vi "Initialization.vi"(6 "Skip Loading?":bool, 7 "Model Name":T3, 8 "Error In":errorcluster, 9 "Intialize?":bool=TRUE, 10 "Inputs":T1, 11 "Start SM":dbl=100.0 format="%#_13g") -> (0 "error out":errorcluster, 1 "Completed":bool, 4 "Status":cluster{"Status":string, "Elapsed Time":dbl}, 5 "Waveform Graph":dbl[][](graph))   [LabVIEW 2017]
doc: "Changelog:\n\n------------\nv0.1:\n- Bypass sensor 1 for all front\n\nv0.1:\n- Start Travel time taken from when the start moving command is given (previous state)\n- Total travel time is taken until the movement is stopped"
uses:
  controls/Model Name.ctl
  controls/All Inputs.ctl
  controls/SACB DI.ctl
  controls/Initialization.ctl
  controls/FGV DO.ctl
panel:
  in  "Stall Time":u32=100
  out "Graph":dbl[][](array[numeric])
  in  "Delay (for Rest)":u32=100
  in  "Timeout (ms)":u32=45000
  # "Inputs"
  # "Variables"
  # "Outputs"
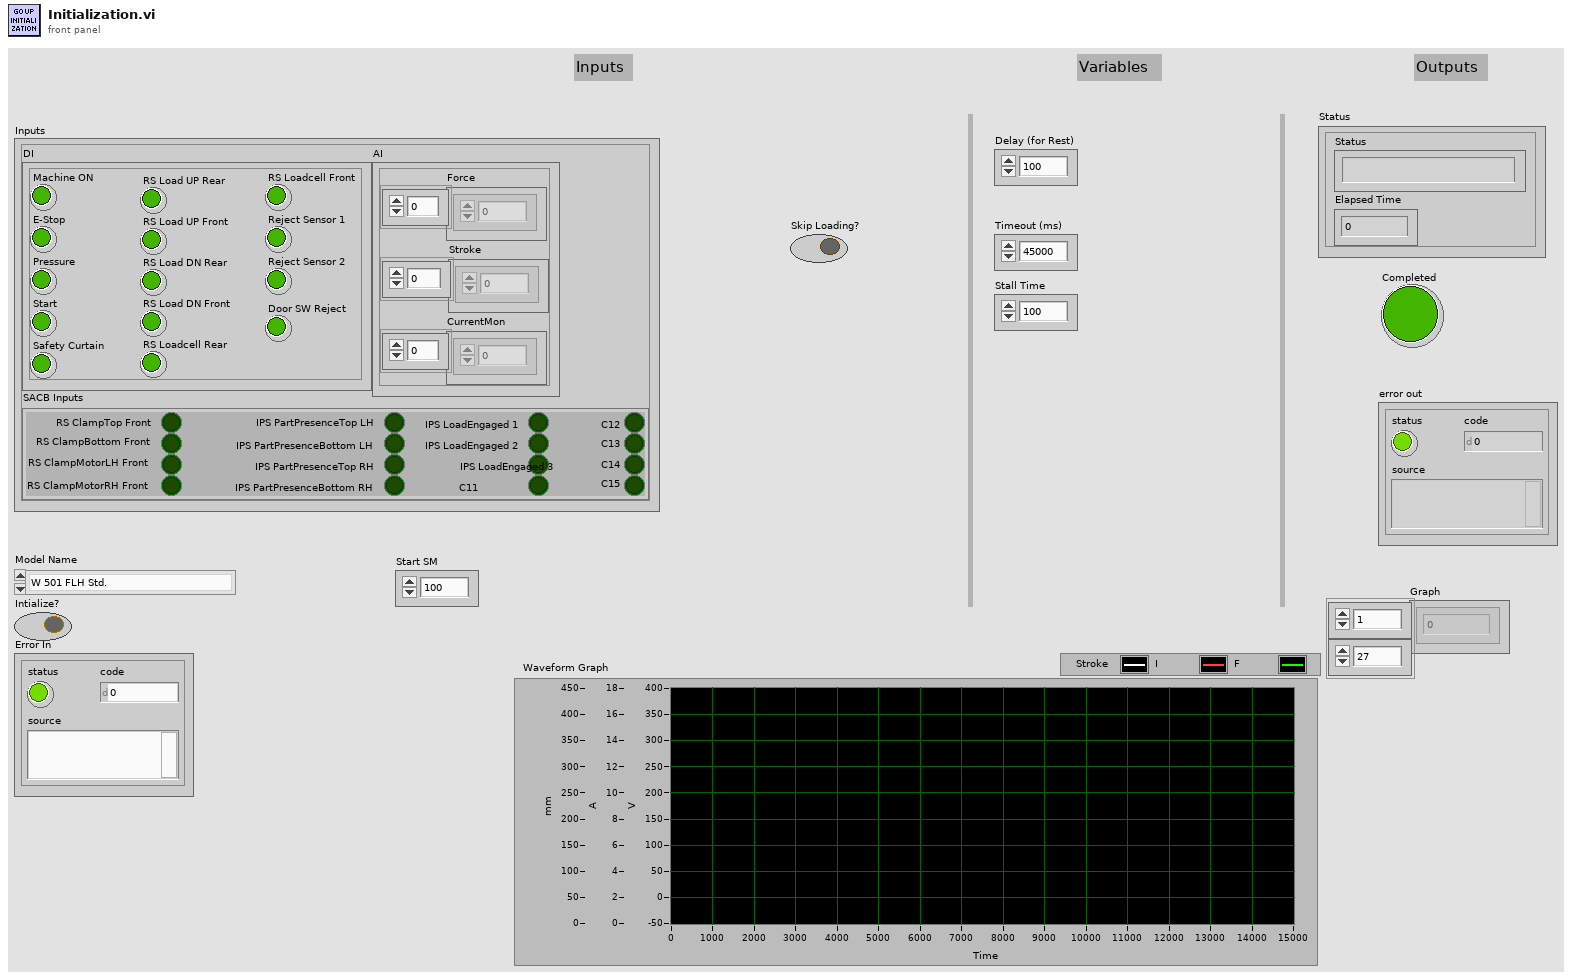
[diagram p1: front panel]
types:
  T1 = typedef "All Inputs.ctl" = cluster{"DI":cluster{"Machine ON":bool, "E-Stop":bool, "Pressure":bool, "Start":bool, "Safety Curtain":bool, "RS Load UP Rear":bool, "RS Load UP Front":bool, "RS Load DN Rear":bool, "RS Load DN Front":bool, "RS Loadcell Rear":bool, "RS Loadcell Front":bool, "Reject Sensor 1":bool, "Reject Sensor 2":bool, "Door SW Reject":bool}, "AI":cluster{"Force":dbl[], "Stroke":dbl[], "CurrentMon":dbl[]}, "SACB Inputs":T2}
  T2 = typedef "SACB DI.ctl" = cluster{"RS ClampTop Front":bool, "RS ClampBottom Front":bool, "RS ClampMotorLH Front":bool, "RS ClampMotorRH Front":bool, "IPS PartPresenceTop LH":bool, "IPS PartPresenceBottom LH":bool, "IPS PartPresenceTop RH":bool, "IPS PartPresenceBottom RH":bool, "IPS LoadEngaged 1":bool, "IPS LoadEngaged 2":bool, "IPS LoadEngaged 3":bool, "C11":bool, "C12":bool, "C13":bool, "C14":bool, "C15":bool}
  T3 = typedef "Model Name.ctl" = enum16{"W 501 FLH Std.", "W 501 FRH Std.", "W 601 FR RH Std", "W 601 FR LH Std", "W 601 RR RH Std", "W 601 RR LH Std", "W 601 FR RH AP", "W 601 FR LH AP", "W 601 RR RH AP", "W 601 RR LH AP"}
  T4 = typedef "Initialization.ctl" = enum16{"Initialize", "Check SM Position", "Check Bottom Position", "Go UP", "Check for Stall", "Turn Off Supply", "Wait for Rest", "Stall for 1s", "Turn off Supply 2", "Wait for BDC", "Done", "Error"}
  T5 = typedef "FGV DO.ctl" = enum16{"Initialize", "Start Task", "Clamping", "Load CYL", "Contactors", "Loadcell CYL", "BSL", "Read DO", "Clear Tasks", "Clear Task"}
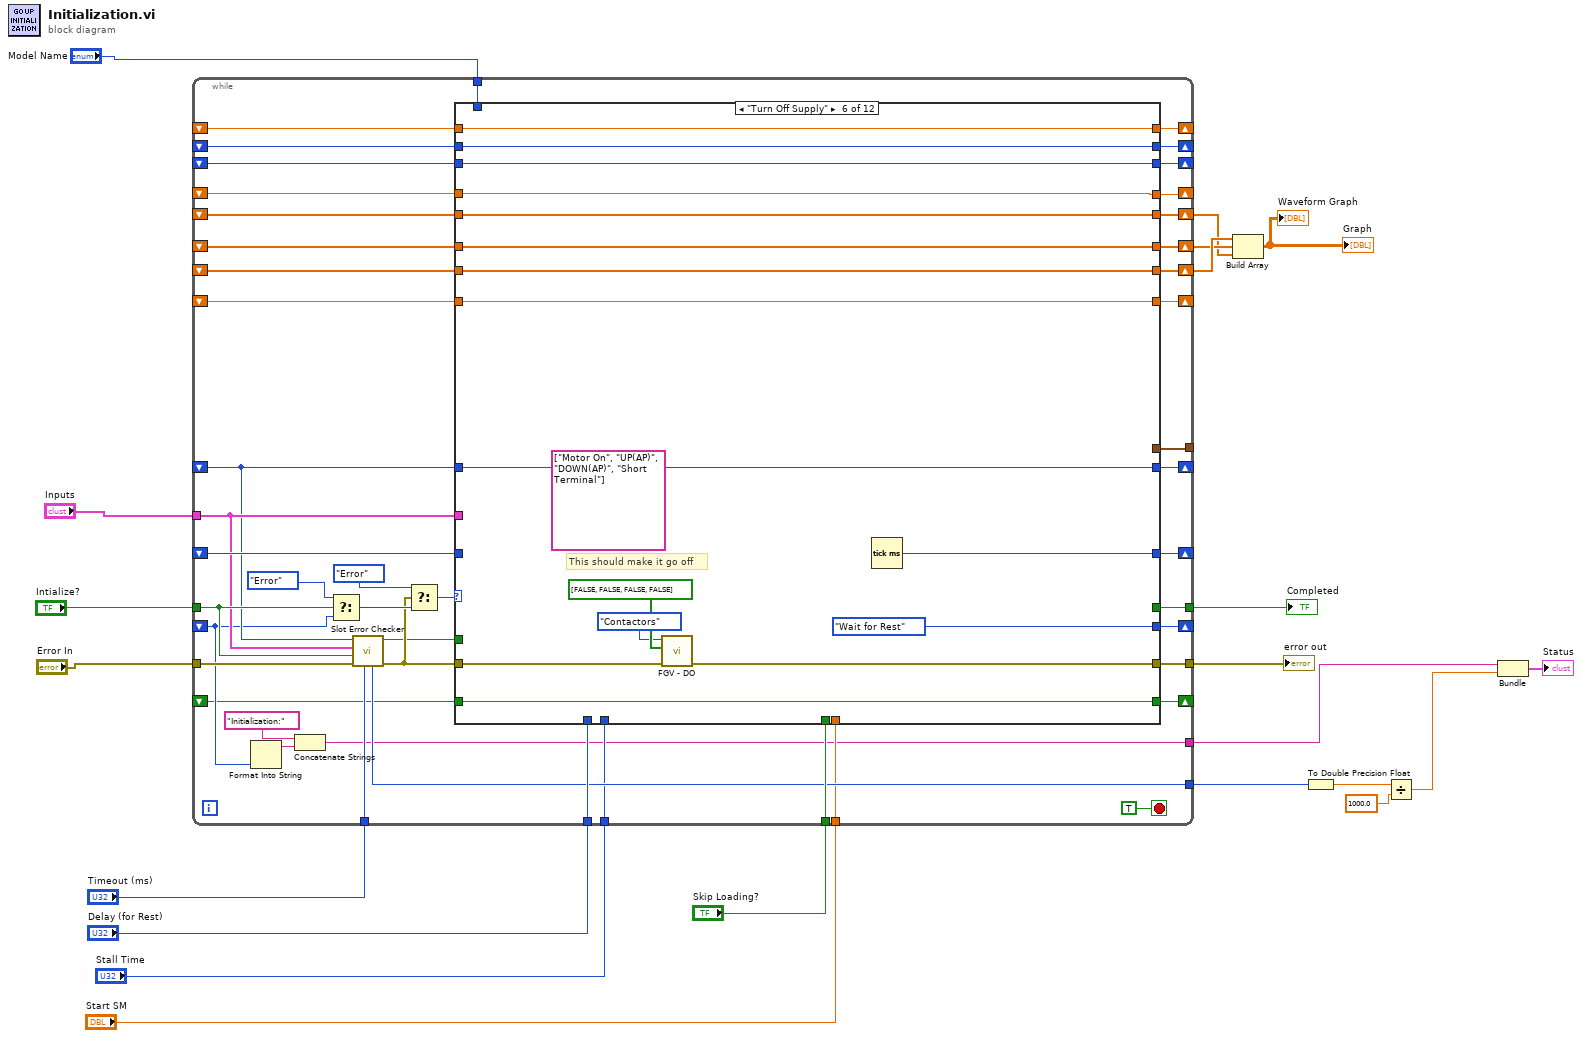
[diagram p0: block diagram]
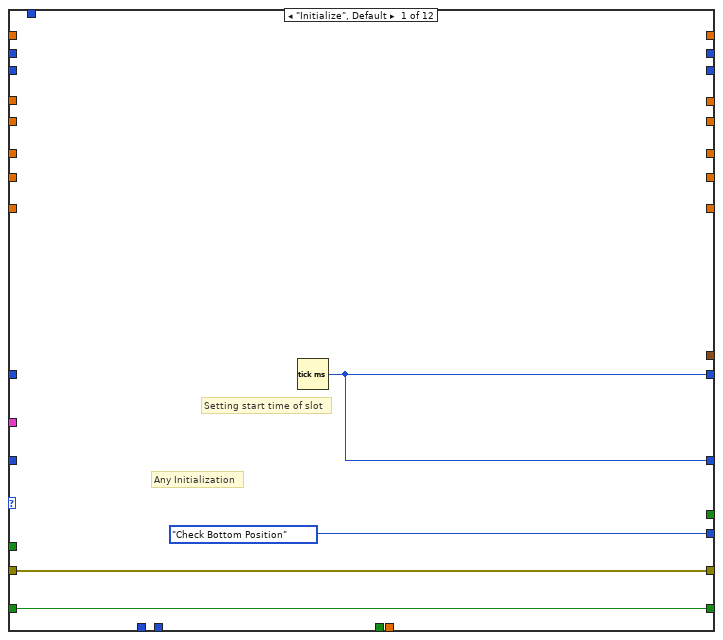
[diagram p2: hidden frame]
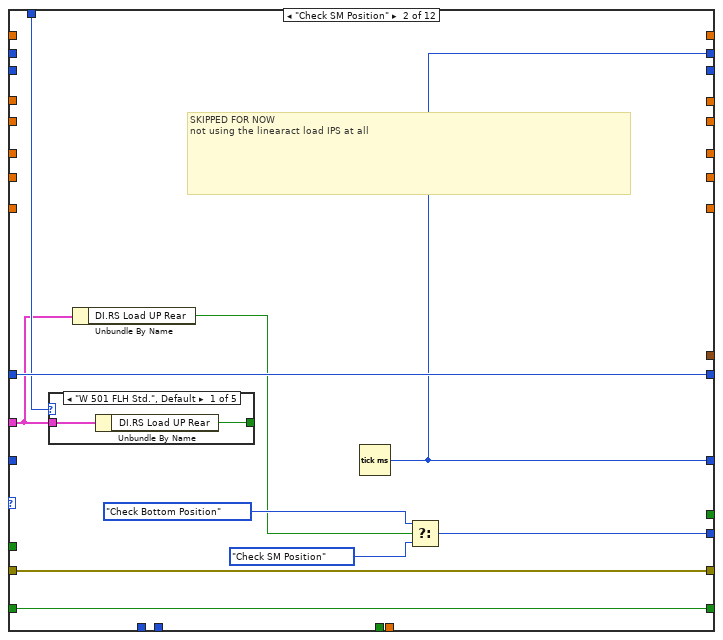
[diagram p3: hidden frame]
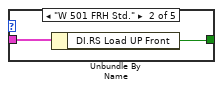
[diagram p4: hidden frame]
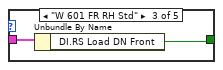
[diagram p5: hidden frame]
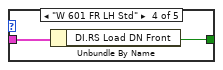
[diagram p6: hidden frame]
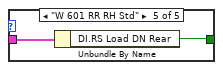
[diagram p7: hidden frame]
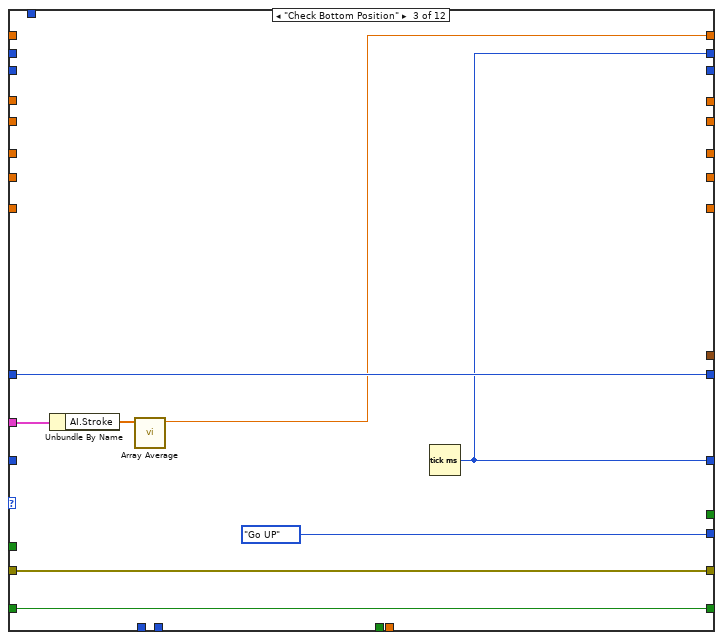
[diagram p8: hidden frame]
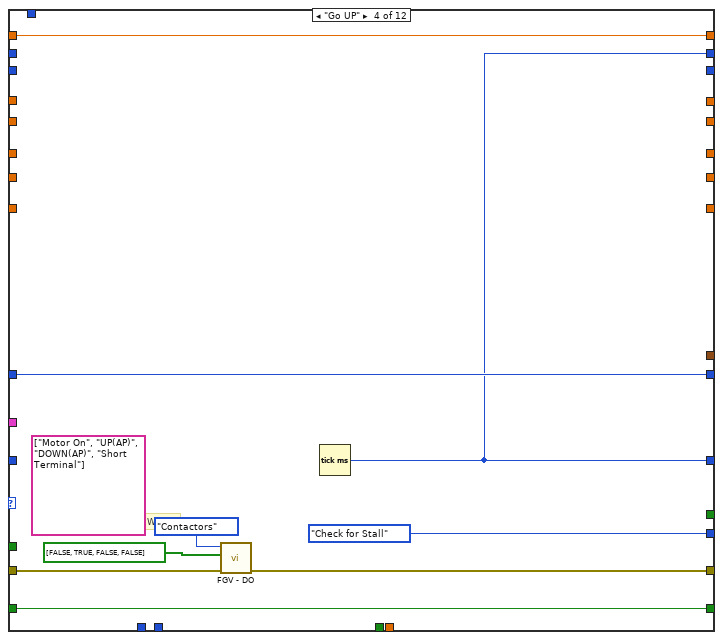
[diagram p9: hidden frame]
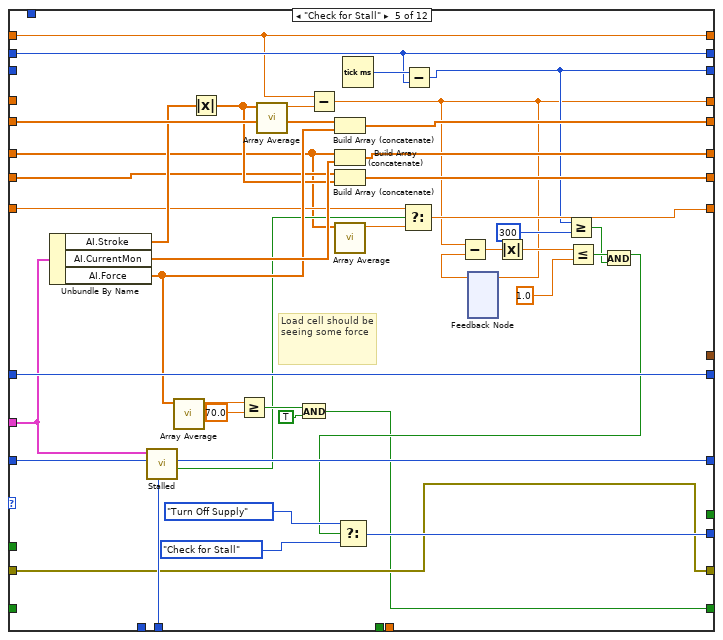
[diagram p10: hidden frame]
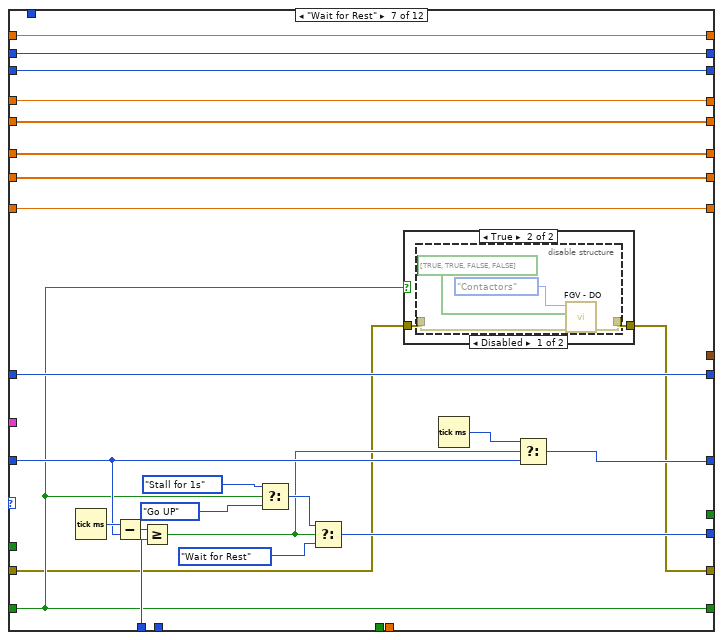
[diagram p11: hidden frame]
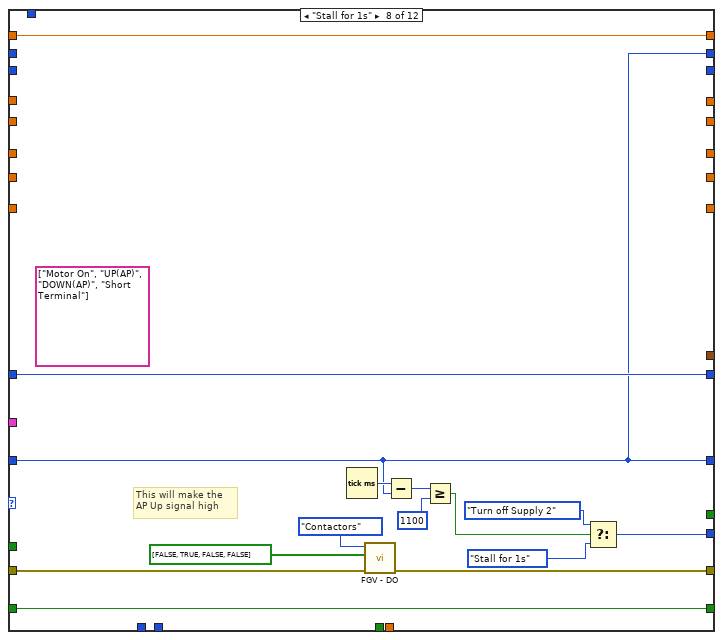
[diagram p14: hidden frame]
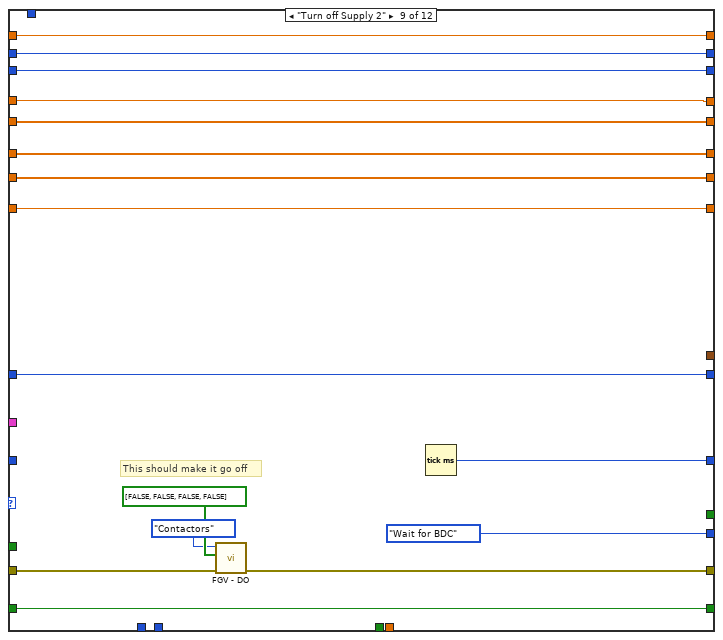
[diagram p15: hidden frame]
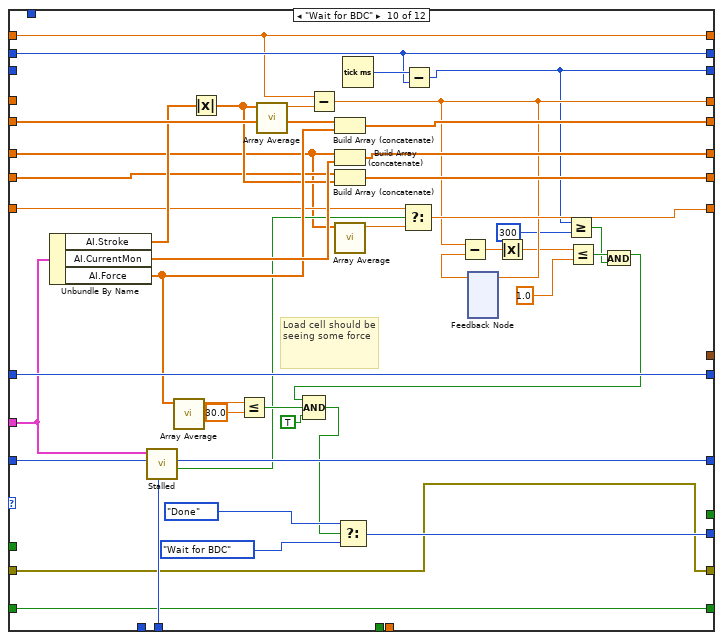
[diagram p16: hidden frame]
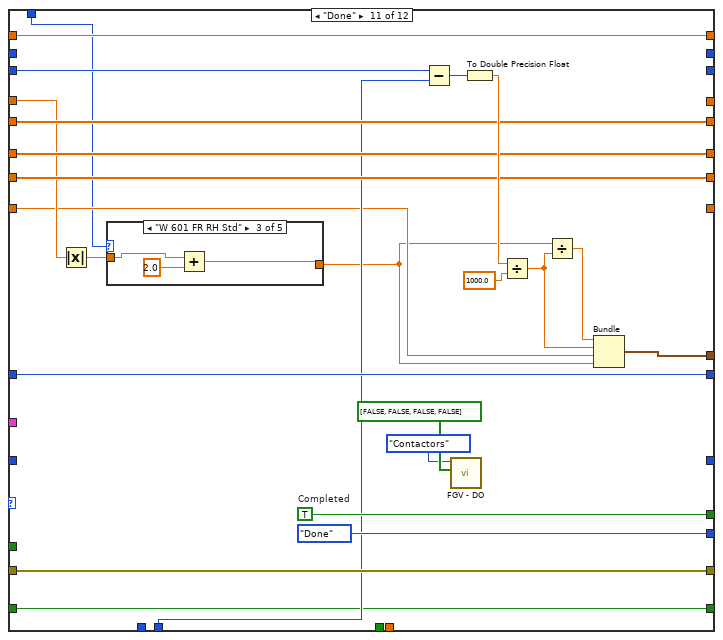
[diagram p17: hidden frame]
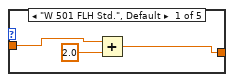
[diagram p18: hidden frame]
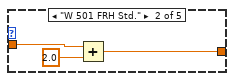
[diagram p19: hidden frame]
diagram:
  n1 = while {
    tunnel: "Intialize?" -> [w60]
    shift-right: [w67] -> _
    shift-left: _ -> [w29]
    shift-right: [w66] -> _
    shift-left: _ -> [w65]
    tunnel: "Error In" -> [w61]
    tunnel: [w64] -> w21
    tunnel: [w63] -> w20
    tunnel: "Inputs" -> [w59]
    shift-right: [w62] -> _
    shift-left: _ -> [w58]
    tunnel: "Delay (for Rest)" -> [w55]
    tunnel: "Timeout (ms)" -> [w54]
    tunnel: "Model Name" -> [w53]
    shift-right: [w52] -> _
    shift-left: _ -> [w51]
    shift-right: [w50] -> w11
    shift-left: _ -> [w49]
    shift-right: [w48] -> _
    shift-left: _ -> [w47]
    tunnel: [w46] -> _
    tunnel: "Skip Loading?" -> [w45]
    tunnel: [w44] -> w12
    shift-right: [w42] -> _
    shift-left: _ -> [w41]
    shift-right: [w40] -> w10
    shift-left: _ -> [w39]
    shift-right: [w38] -> w8
    shift-left: _ -> [w37]
    shift-right: [w36] -> _
    shift-left: _ -> [w35]
    tunnel: "Stall Time" -> [w34]
    tunnel: "Start SM" -> [w32]
    tunnel: [w28] -> w5
    shift-right: [w26] -> _
    shift-left: _ -> [w27]
    shift-right: [w25] -> _
    shift-left: _ -> [w24]
    stop <- TRUE stop-if-true
    n2 = Format Into String(w29) -> (resulting string=w31:string)  [unwired: 3 in, 1 out]
    n3 = Concatenate Strings("Initialization:", w31) -> (w28:string)
    n4 = Select(t=Initialization."Error", s=w60, f=w29) -> (s? t:f=w57:T4)
    n5 = call "Slot Error Checker.vi"("Timeout (ms)"=w54, "error in (no error)"=w61, "Intialize?"=w60, "Inputs"=w59, "start time"=w58) -> ("error out"=w56:errorcluster, "Safety Interrupt?"=w33:bool, "Slot Time"=w44:u32)  [unwired: 4 in]
    n6 = Select(t=Initialization."Error", s=w56, f=w57) -> (s? t:f=w43:T4)
    n7 = case shown="\"Turn Off Supply\"" w43 {
      tunnel: [Initialization."Check Bottom Position" w80 Initialization."Go UP" Initialization."Check for Stall" w147 Initialization."Wait for Rest" w189 w203 Initialization."Wait for BDC" w269 Initialization."Done" Initialization."Done"] -> w67
      tunnel: [w70 w77 w94 w102 w140 w165 w174 w206 w228 w262 _ _] -> w66
      tunnel: w65 -> [_ _ _ _ w150 _ w175 w206 _ w272 _ _]
      tunnel: w56 -> [w71 w82 w99 w109 w128 w167 w171 w214 w230 w250 w296 w322]
      tunnel: [w71 w82 w99 w108 w128 w156 w170 w213 w219 w250 w296 w322] -> w64
      tunnel: [_ _ _ _ _ _ _ _ _ _ w295 TRUE ("Completed")] -> w63
      tunnel: w59 -> [_ w75 w96 _ w146 _ _ _ _ w268 _ _]
      tunnel: [w70 w81 w100 w106 w151 w164 w188 w211 w227 w273 w294 w319] -> w62
      tunnel: w58 -> [_ w81 w100 w106 w151 w164 w188 w211 w227 w273 w294 w319]
      tunnel: w55 -> [_ _ _ _ _ _ w187 _ _ _ _ _]
      tunnel: w53 -> [_ w76 _ _ _ _ _ _ _ _ w277 _]
      tunnel: [_ w77 w94 w102 w139 w161 w184 w206 w224 w261 _ _] -> w52
      tunnel: w51 -> [_ _ _ _ w139 w161 w184 _ w224 w261 _ _]
      tunnel: [_ _ _ _ w141 w163 w186 _ w226 w263 w288 w312] -> w50
      tunnel: w49 -> [_ _ _ _ w127 w163 w186 _ w226 w249 w288 w312]
      tunnel: [_ _ _ _ w117 w162 w185 _ w225 w238 _ _] -> w48
      tunnel: w47 -> [_ _ _ _ _ w162 w185 _ w225 _ w284 _]
      tunnel: [_ _ _ _ _ _ _ _ _ _ w289 _] -> w46
      tunnel: w45 -> [_ _ _ _ _ _ _ _ _ _ _ _]
      tunnel: [_ _ w95 w105 w130 w160 w183 w210 w223 w252 w286 w318] -> w42
      tunnel: w41 -> [_ _ _ w105 w130 w160 w183 w210 w223 w252 w286 w318]
      tunnel: [_ _ _ _ w143 w158 w180 _ w221 w265 w287 w311] -> w40
      tunnel: w39 -> [_ _ _ _ w123 w158 w180 _ w221 w245 w287 w311]
      tunnel: [_ _ _ _ w142 w159 w181 _ w222 w264 w285 w310] -> w38
      tunnel: w37 -> [_ _ _ _ w134 w159 w181 _ w222 w256 w285 w310]
      tunnel: [_ _ _ _ w111 w157 w182 _ w220 w243 _ _] -> w36
      tunnel: w35 -> [_ _ _ _ _ w157 w182 _ w220 _ w281 _]
      tunnel: w34 -> [_ _ _ _ w133 _ _ _ _ w255 w282 _]
      tunnel: w33 -> [_ _ _ _ _ _ _ _ _ _ _ w313]
      tunnel: w32 -> [_ _ _ _ _ _ _ _ _ _ _ _]
      tunnel: [_ _ _ _ w124 w155 w179 _ w218 w246 _ _] -> w26
      tunnel: w27 -> [_ _ _ _ w125 w155 w179 _ w218 w247 w278 _]
      tunnel: [w69 w73 w93 w101 w113 w154 w172 w208 w217 w234 w274 w309] -> w25
      tunnel: w24 -> [w69 w73 w93 w101 _ w154 w172 w208 w217 w234 w274 w309]
      frame "Initialize", Default {
        # "Setting start time of slot"
        # "Any Initialization"
        n8 = Tick Count (ms)() -> (millisecond timer value=w70:u32)
      }
      frame "Check SM Position" {
        # "SKIPPED FOR NOW \nnot using the linearact load IPS at all"
        n9 = case shown="\"W 501 FLH Std.\", Default" w76 {
          tunnel: w75 -> [w83 w86 w88 w89 w92]
          tunnel: [w84 w85 w87 w90 w91] -> _
          frame "W 501 FLH Std.", Default {
            n10 = Unbundle By Name(w83) -> ("DI.RS Load UP Rear"=w84:bool)
          }
          frame "W 501 FRH Std." {
            n11 = Unbundle By Name(w86) -> ("DI.RS Load UP Front"=w85:bool)
          }
          frame "W 601 FR RH Std" {
            n12 = Unbundle By Name(w88) -> ("DI.RS Load DN Front"=w87:bool)
          }
          frame "W 601 FR LH Std" {
            n13 = Unbundle By Name(w89) -> ("DI.RS Load DN Front"=w90:bool)
          }
          frame "W 601 RR RH Std" {
            n14 = Unbundle By Name(w92) -> ("DI.RS Load DN Rear"=w91:bool)
          }
        }
        n15 = Unbundle By Name(w75) -> ("DI.RS Load UP Rear"=w74:bool)
        n16 = Tick Count (ms)() -> (millisecond timer value=w77:u32)
        n17 = Select(t=Initialization."Check Bottom Position", s=w74, f=Initialization."Check SM Position") -> (s? t:f=w80:T4)
      }
      frame "Check Bottom Position" {
        n18 = Unbundle By Name(w96) -> ("AI.Stroke"=w97:dbl[])
        n19 = call "Array Average.vi"("data"=w97) -> ("Numeric"=w95:dbl)  [unwired: 10 in]
        n20 = Tick Count (ms)() -> (millisecond timer value=w94:u32)
      }
      frame "Go UP" {
        (unwired) string[] ["Motor On", "UP(AP)", "DOWN(AP)", "Short Terminal"]
        # "Changes According to WR"
        n21 = call "FGV - DO.vi"("error in"=w109, "Digital Outs"=bool[] [FALSE, TRUE, FALSE, FALSE], "State"=FGV_DO."Contactors") -> ("error out"=w108:errorcluster)  [unwired: 7 in, 1 out]
        n22 = Tick Count (ms)() -> (millisecond timer value=w102:u32)
      }
      frame "Check for Stall" {
        # "Load cell should be seeing some force"
        n23 = Unbundle By Name(w146) -> ("AI.Stroke"=w132:dbl[], "AI.CurrentMon"=w144:dbl[], "AI.Force"=w136:dbl[])
        n24 = call "Stalled.vi"("Stall Time (ms)"=w133, "millisecond timer value in"=w150, "Inputs"=w146) -> ("Stalled"=w126:bool, "millisecond timer value out"=w140:u32)  [unwired: 7 in]
        n25 = call "Array Average.vi"("data"=w136) -> ("Numeric"=w135:dbl)  [unwired: 10 in]
        n26 = Absolute Value(x=w132) -> (abs(x)=w131:dbl[])
        n27 = Greater Or Equal?(x=w135, y=70.0) -> (x >= y?=w137:bool)
        n28 = call "Array Average.vi"("data"=w131) -> ("Numeric"=w129:dbl)  [unwired: 10 in]
        n29 = And(x=w137, y=TRUE) -> (x .and. y?=w113:bool)
        n30 = Subtract(x=w130, y=w129) -> (x-y=w111:dbl)
        n31 = Build Array (concatenate)(w134, w136) -> (w142:dbl[])
        n32 = Build Array (concatenate)(w123, w144) -> (w143:dbl[])
        n33 = Build Array (concatenate)(w127, w131) -> (w141:dbl[])
        n34 = call "Array Average.vi"("data"=w123) -> ("Numeric"=w122:dbl)  [unwired: 10 in]
        n35 = Tick Count (ms)() -> (millisecond timer value=w145:u32)
        n36 = Select(t=w125, s=w126, f=w122) -> (s? t:f=w124:dbl)
        n37 = Subtract(x=w145, y=w139) -> (x-y=w117:u32)
        n38 = feedback #1() -> (w121:dbl)  [unwired: 1 in]
        n39 = Subtract(x=w111, y=w121) -> (x-y=w120:dbl)
        n40 = feedback-in #1(w111) -> ()
        n41 = Absolute Value(x=w120) -> (abs(x)=w112:dbl)
        n42 = Greater Or Equal?(x=w117, y=u32 300) -> (x >= y?=w114:bool)
        n43 = Less Or Equal?(x=w112, y=1.0) -> (x <= y?=w118:bool)
        n44 = And(x=w118, y=w114) -> (x .and. y?=w115:bool)
        n45 = Select(t=Initialization."Turn Off Supply", s=w115, f=Initialization."Check for Stall") -> (s? t:f=w147:T4)
      }
      frame "Turn Off Supply" {
        (unwired) string[] ["Motor On", "UP(AP)", "DOWN(AP)", "Short Terminal"]
        # "This should make it go off"
        n46 = call "FGV - DO.vi"("error in"=w167, "Digital Outs"=bool[] [FALSE, FALSE, FALSE, FALSE], "State"=FGV_DO."Contactors") -> ("error out"=w156:errorcluster)  [unwired: 7 in, 1 out]
        n47 = Tick Count (ms)() -> (millisecond timer value=w165:u32)
      }
      frame "Wait for Rest" {
        n48 = Tick Count (ms)() -> (millisecond timer value=w191:u32)
        n49 = Subtract(x=w191, y=w175) -> (x-y=w190:u32)
        n50 = Greater Or Equal?(x=w190, y=w187) -> (x >= y?=w173:bool)
        n51 = Select(t=Initialization."Stall for 1s", s=w172, f=Initialization."Go UP") -> (s? t:f=w177:T4)
        n52 = Select(t=w177, s=w173, f=Initialization."Wait for Rest") -> (s? t:f=w189:T4)
        n53 = case shown="True" w172 {
          tunnel: w171 -> [w192 w194]
          tunnel: [w192 w193] -> w170
          frame False {
          }
          frame True {
            n54 = disable-structure shown="Disabled" {
              disable-tunnel: w194 -> [w197 w199]
              disable-tunnel: [w196 w199] -> w193
              frame Disabled {
                n55 = call "FGV - DO.vi"("error in"=w197, "Digital Outs"=bool[] [TRUE, TRUE, FALSE, FALSE], "State"=FGV_DO."Contactors") -> ("error out"=w196:errorcluster)  [unwired: 7 in, 1 out]
              }
              frame Enabled {
              }
            }
          }
        }
        n56 = Tick Count (ms)() -> (millisecond timer value=w176:u32)
        n57 = Select(t=w176, s=w173, f=w175) -> (s? t:f=w174:u32)
      }
      frame "Stall for 1s" {
        (unwired) string[] ["Motor On", "UP(AP)", "DOWN(AP)", "Short Terminal"]
        # "This will make the  \nAP Up signal high"
        n58 = Tick Count (ms)() -> (millisecond timer value=w207:u32)
        n59 = call "FGV - DO.vi"("error in"=w214, "Digital Outs"=bool[] [FALSE, TRUE, FALSE, FALSE], "State"=FGV_DO."Contactors") -> ("error out"=w213:errorcluster)  [unwired: 7 in, 1 out]
        n60 = Subtract(x=w207, y=w206) -> (x-y=w202:u32)
        n61 = Greater Or Equal?(x=w202, y=u32 1100) -> (x >= y?=w200:bool)
        n62 = Select(t=Initialization."Turn off Supply 2", s=w200, f=Initialization."Stall for 1s") -> (s? t:f=w203:T4)
      }
      frame "Turn off Supply 2" {
        # "This should make it go off"
        n63 = call "FGV - DO.vi"("error in"=w230, "Digital Outs"=bool[] [FALSE, FALSE, FALSE, FALSE], "State"=FGV_DO."Contactors") -> ("error out"=w219:errorcluster)  [unwired: 7 in, 1 out]
        n64 = Tick Count (ms)() -> (millisecond timer value=w228:u32)
      }
      frame "Wait for BDC" {
        # "Load cell should be seeing some force"
        n65 = Unbundle By Name(w268) -> ("AI.Stroke"=w254:dbl[], "AI.CurrentMon"=w266:dbl[], "AI.Force"=w258:dbl[])
        n66 = call "Stalled.vi"("Stall Time (ms)"=w255, "millisecond timer value in"=w272, "Inputs"=w268) -> ("Stalled"=w248:bool, "millisecond timer value out"=w262:u32)  [unwired: 7 in]
        n67 = call "Array Average.vi"("data"=w258) -> ("Numeric"=w257:dbl)  [unwired: 10 in]
        n68 = Absolute Value(x=w254) -> (abs(x)=w253:dbl[])
        n69 = Less Or Equal?(x=w257, y=30.0) -> (x <= y?=w259:bool)
        n70 = call "Array Average.vi"("data"=w253) -> ("Numeric"=w251:dbl)  [unwired: 10 in]
        n71 = Subtract(x=w252, y=w251) -> (x-y=w243:dbl)
        n72 = Build Array (concatenate)(w256, w258) -> (w264:dbl[])
        n73 = Build Array (concatenate)(w245, w266) -> (w265:dbl[])
        n74 = Build Array (concatenate)(w249, w253) -> (w263:dbl[])
        n75 = call "Array Average.vi"("data"=w245) -> ("Numeric"=w244:dbl)  [unwired: 10 in]
        n76 = Tick Count (ms)() -> (millisecond timer value=w267:u32)
        n77 = Select(t=w247, s=w248, f=w244) -> (s? t:f=w246:dbl)
        n78 = Subtract(x=w267, y=w261) -> (x-y=w238:u32)
        n79 = feedback #2() -> (w242:dbl)  [unwired: 1 in]
        n80 = Subtract(x=w243, y=w242) -> (x-y=w241:dbl)
        n81 = feedback-in #2(w243) -> ()
        n82 = Absolute Value(x=w241) -> (abs(x)=w235:dbl)
        n83 = Greater Or Equal?(x=w238, y=u32 300) -> (x >= y?=w236:bool)
        n84 = Less Or Equal?(x=w235, y=1.0) -> (x <= y?=w239:bool)
        n85 = And(x=w239, y=w236) -> (x .and. y?=w232:bool)
        n86 = Compound Arithmetic op=AND(w232, w259, TRUE) -> (w233:bool)
        n87 = Select(t=Initialization."Done", s=w233, f=Initialization."Wait for BDC") -> (s? t:f=w269:T4)
      }
      frame "Done" {
        w295 = TRUE  # Completed
        n88 = Absolute Value(x=w281) -> (abs(x)=w276:dbl)
        n89 = case shown="\"W 601 FR RH Std\"" w277 {
          tunnel: w276 -> [w299 w302 w305 w307 w308]
          tunnel: [w298 w301 w304 w307 w308] -> w275
          frame "W 501 FLH Std.", Default {
            n90 = Add(x=w299, y=2.0) -> (x+y=w298:dbl)
          }
          frame "W 501 FRH Std." {
            n91 = Add(x=w302, y=2.0) -> (x+y=w301:dbl)
          }
          frame "W 601 FR RH Std" {
            n92 = Add(x=w305, y=2.0) -> (x+y=w304:dbl)
          }
          frame "W 601 FR LH Std" {
          }
          frame "W 601 RR RH Std" {
          }
        }
        n93 = Subtract(x=w284, y=w282) -> (x-y=w283:u32)
        n94 = call "FGV - DO.vi"("Digital Outs"=bool[] [FALSE, FALSE, FALSE, FALSE], "State"=FGV_DO."Contactors") -> ()  [unwired: 8 in, 2 out]
        n95 = To Double Precision Float(number=w283) -> (double precision float=w292:dbl)
        n96 = Divide(x=w292, y=1000.0) -> (x/y=w290:dbl)
        n97 = Divide(x=w275, y=w290) -> (x/y=w291:dbl)
        n98 = Bundle(w291, w290, "Numeric"=w278, w275) -> (w289:cluster{dbl, dbl, "Numeric":dbl, dbl})  [unwired: 1 in]
      }
      frame "Error" {
        w314 = T5[] [enum."Contactors", enum."Loadcell CYL"] items=["Initialize", "Start Task", "Clamping", "Load CYL", "Contactors", "Loadcell CYL", "BSL", "Read DO", "Clear Tasks", "Clear Task"]
        w316 = T5[] [enum."Clamping", enum."Contactors", enum."Loadcell CYL"] items=["Initialize", "Start Task", "Clamping", "Load CYL", "Contactors", "Loadcell CYL", "BSL", "Read DO", "Clear Tasks", "Clear Task"]
        n99 = Select(t=w316, s=w313, f=w314) -> (s? t:f=w315:T5[])
        n100 = for {
          tunnel: w315 -> [w324] mode=indexing
          tunnel: bool[] [FALSE, FALSE, FALSE, FALSE] ("Digital Outs") -> [w323]
          n101 = call "FGV - DO.vi"("Digital Outs"=w323, "State"=w324) -> ()  [unwired: 8 in, 2 out]
        }
      }
    }
  }
  "error out" <- w21
  "Completed" <- w20
  n102 = Build Array(w11, w10, w8) -> (→"Graph" →"Waveform Graph":dbl[][])
  n103 = To Double Precision Float(number=w12) -> (double precision float=w16:dbl)
  n104 = Divide(x=w16, y=1000.0) -> (x/y=w14:dbl)
  n105 = Bundle(w5, w14) -> (→"Status":cluster{string, dbl})  [unwired: 1 in]
